vi "QPNRDecode.vi"(11 "String":string) -> (3 "PhaseNoise":dbl)   [LabVIEW 2017, in "SARemote.lvlib"]
uses:
  SARemote.lvlib
panel:
  out "match substring 3":string
  out "output cluster":T1
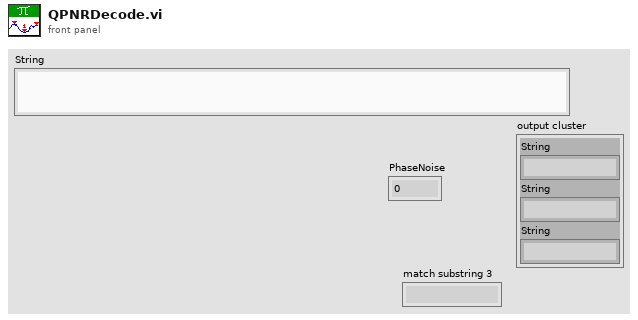
[diagram p1: front panel]
types:
  T1 = cluster{"String":string, "String":string, "String":string}
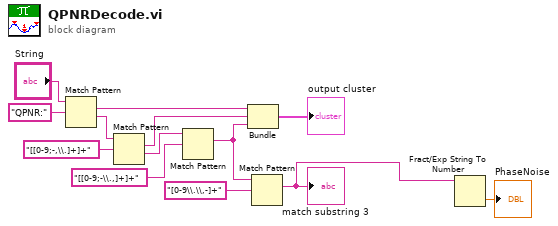
[diagram p0: block diagram]
diagram:
  n1 = Match Pattern(string="String", regular expression="QPNR:") -> (match substring=w7:string, after substring=w11:string)  [unwired: 1 in, 2 out]
  n2 = Match Pattern(string=w11, regular expression="[[0-9;-,\\.]+]+") -> (match substring=w6:string, after substring=w8:string)  [unwired: 1 in, 2 out]
  n3 = Match Pattern(string=w8, regular expression="[[0-9;-\\.,]+]+") -> (match substring=w4:string)  [unwired: 1 in, 3 out]
  n4 = Bundle("String"=w7, "String"=w6, "String"=w4) -> (→"output cluster":T1)  [unwired: 1 in]
  n5 = Match Pattern(string=w4, regular expression="[0-9\\.\\,-]+") -> (match substring=w2:string)  [unwired: 1 in, 3 out]
  "match substring 3" <- w2
  n6 = Fract/Exp String To Number(string=w2) -> (number=→"PhaseNoise":dbl)  [unwired: 3 in, 1 out]
